vi "rsscope Initialize with Options.vi"(0 "VISA resource name":refnum<visa-resource-name>="TCPIP::192.168.5.120::INST", 2 "Option string (\"\")":string, 5 "ID Query (T: Check)":bool=TRUE, 7 "Reset (T: Reset)":bool=TRUE, 11 "error in (no error)":errorcluster) -> (4 "VISA resource name out":refnum<visa-resource-name>, 15 "error out":errorcluster)   [LabVIEW 2018]
doc: "This VI opens a new session to the instrument.\nCompared to the <b>Initialize.vi</b>, this one allows for additional settings in the <b>Option string</b>."
uses:
  _utility/rsidr_core.llb/type_Session_Parameter_int32.ctl
  _utility/rsscope_core_global.vi
  _utility/rsidr_core.llb/rsscope_rsidr_core.lvlib
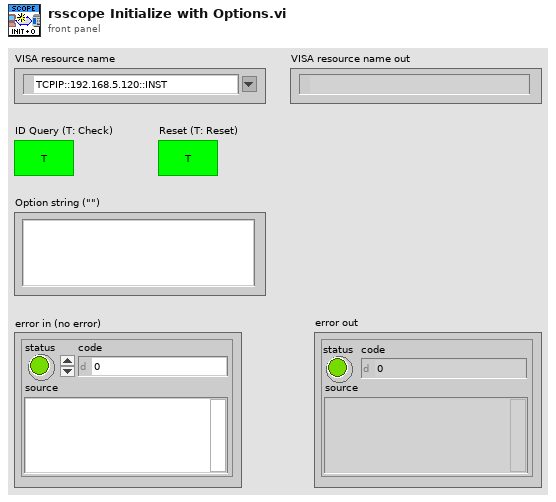
[diagram p1: front panel]
types:
  T1 = typedef "rsscope_rsidr_core.lvlib/type_Session_Parameter_int32.ctl" = enum16{"OPC Timeout", "Additional Flags", "Wait Before Write", "Wait Before Read", "Bin Data Chunk Size", "VISA Access Mode", "VISA Timeout", "Bin Float Number Format", "Bin Integer Number Format", "STBpollVISAtimeout", "OPCwaitMode"}
  T2 = typedef "rsscope_rsidr_core.lvlib/type_Input_Format_RepCap.ctl" = cluster{"repCapName":string, "indetifiers":string[], "cmdValues":string[]}
  T3 = typedef "rsscope_rsidr_core.lvlib/type_Input_Format_RangeTable.ctl" = cluster{"Type":u16, "Name":string, "Entries":cluster{"Name":string, "Value 1":dbl, "Value 2":dbl, "Command":string}[]}
  T4 = typedef "rsscope_rsidr_core.lvlib/type_Input_Format_Attribute.ctl" = cluster{"Level":i32, "Class Only":bool, "Identifier":string, "Descriptive Name":string, "Data Type":u16, "Command":string, "Access":u16, "Range Table":string, "Read Callback":string, "Write Callback":string, "Supported Models":string, "Instrument Options":string, "Flags":i32, "Help":string}
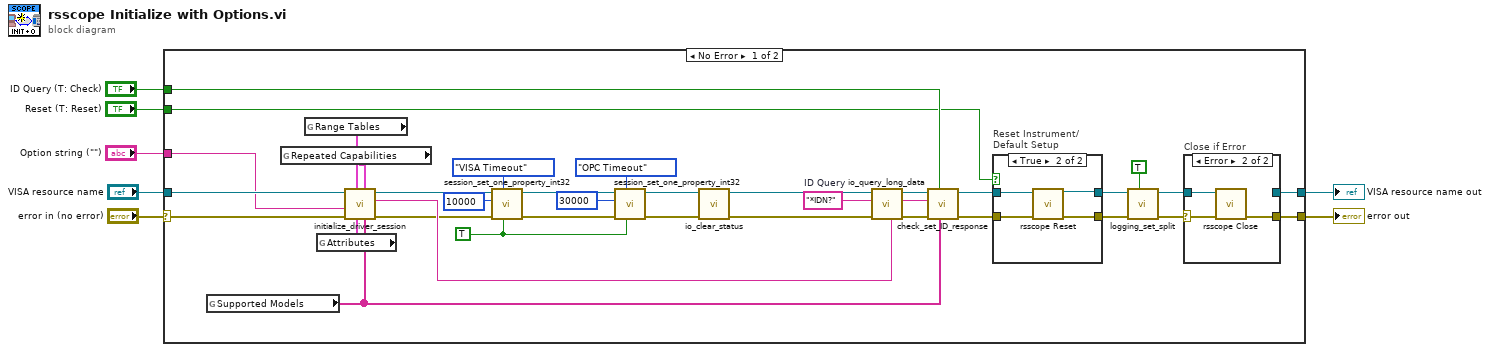
[diagram p0: block diagram]
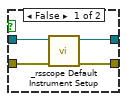
[diagram p3: hidden frame]
diagram:
  n1 = case shown="No Error" "error in (no error)" {
    selector: "error in (no error)" -> [w35 w57]
    tunnel: [w43 _] -> w7
    tunnel: [w36 w57] -> w6
    tunnel: "VISA resource name" -> [w34 _]
    tunnel: "Option string (\"\")" -> [w24 _]
    tunnel: "ID Query (T: Check)" -> [w23 _]
    tunnel: "Reset (T: Reset)" -> [w22 _]
    frame No Error {
      w10 = TRUE ("Skip setting if in option string (F)")
      w37 = "*IDN?"  # ID Query
      n2 = global read "rsscope_core_global.vi" "Supported Models"() -> (w28:string[])
      n3 = global read "rsscope_core_global.vi" "Repeated Capabilities"() -> (w26:T2[])
      n4 = global read "rsscope_core_global.vi" "Range Tables"() -> (w27:T3[])
      n5 = global read "rsscope_core_global.vi" "Attributes"() -> (w25:T4[])
      n6 = call "initialize_driver_session.vi"("Supported instruments"=w28, "Repeated Capabilities"=w26, "Attributes"=w25, "Range Tables"=w27, "error in"=w35, "Option String"=w24, "VISA resource name"=w34) -> ("error out"=w12:errorcluster, "Simulation *IDN? response out"=w21:string, "VISA resource name out"=w11:refnum<visa-resource-name>)  [unwired: 2 in]
      n7 = call "session_set_one_property_int32.vi"("Skip setting if in Options string (F)"=w10, "Session Parameter Integer"=type_Session_Parameter_int32."VISA Timeout" ("Session Parameter to set"), "error in"=w12, "Int32 value in"=10000 ("int32 value in"), "VISA resource name"=w11) -> ("error out"=w17:errorcluster, "VISA resource name out"=w16:refnum<visa-resource-name>)  [unwired: 4 in, 1 out]
      n8 = call "session_set_one_property_int32.vi"("Skip setting if in Options string (F)"=w10, "Session Parameter Integer"=type_Session_Parameter_int32."OPC Timeout" ("Session Parameter to set"), "error in"=w17, "Int32 value in"=30000 ("OPC Timeout"), "VISA resource name"=w16) -> ("error out"=w15:errorcluster, "VISA resource name out"=w14:refnum<visa-resource-name>)  [unwired: 4 in, 1 out]
      n9 = call "io_clear_status.vi"("error in"=w15, "VISA resource name"=w14) -> ("error out"=w9:errorcluster, "VISA resource name out"=w8:refnum<visa-resource-name>)  [unwired: 8 in]
      n10 = call "io_query_long_data.vi"("Simulation read buffer (\"Simulation\")"=w21, "error in"=w9, "write buffer"=w37, "VISA resource name"=w8) -> ("error out"=w40:errorcluster, "read buffer"=w38:string, "VISA resource name out"=w39:refnum<visa-resource-name>)  [unwired: 5 in]
      n11 = call "check_set_ID_response.vi"("Supported instruments in"=w28, "Error if ID Query check fails"=w23, "error in"=w40, "IDN string in"=w38, "VISA resource name"=w39) -> ("error out"=w41:errorcluster, "VISA resource name out"=w42:refnum<visa-resource-name>)  [unwired: 3 in, 2 out]
      n12 = case "Reset Instrument/\nDefault Setup" shown="True" w22 {
        tunnel: w41 -> [w52 w56]
        tunnel: [w50 w55] -> w33
        tunnel: w42 -> [w51 w54]
        tunnel: [w49 w53] -> w32
        frame False {
          n13 = call "_rsscope Default Instrument Setup.vi"("error in (no error)"=w52, "VISA resource name"=w51) -> ("error out"=w50:errorcluster, "VISA resource name out"=w49:refnum<visa-resource-name>)  [unwired: 8 in]
        }
        frame True {
          n14 = call "rsscope Reset.vi"("VISA resource name"=w54, "error in (no error)"=w56) -> ("VISA resource name out"=w53:refnum<visa-resource-name>, "error out"=w55:errorcluster)  [unwired: 12 in]
        }
      }
      n15 = call "logging_set_split.vi"("Evaluate section error (F)"=TRUE, "error in"=w33, "VISA resource name"=w32) -> ("error out"=w31:errorcluster, "VISA resource name out"=w30:refnum<visa-resource-name>)  [unwired: 7 in]
      n16 = case "Close if Error" shown="Error" w31 {
        selector: w31 -> [w44 w47]
        tunnel: w30 -> [w45 w48]
        tunnel: [w45 _] -> w43
        tunnel: [w44 w46] -> w36
        frame No Error {
        }
        frame Error {
          n17 = call "rsscope Close.vi"("error in (no error)"=w47, "VISA resource name"=w48) -> ("error out"=w46:errorcluster)  [unwired: 9 in]
        }
      }
    }
    frame Error {
    }
  }
  "VISA resource name out" <- w7
  "error out" <- w6
